vi "Control Type.vi"(11 "Valve in":refnum<class "InterlockControl.lvclass">) -> (2 "Valve Type":string)   [LabVIEW 2020, in "VolatusControl.lvlib" / "InterlockControl.lvclass"]
uses:
  InterlockControl.lvclass
  InterlockControl.lvclass/InterlockControl.ctl
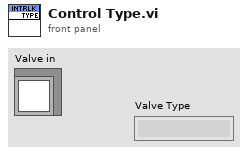
[diagram p1: front panel]
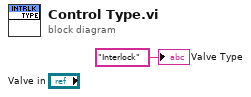
[diagram p0: block diagram]
diagram:
  "Valve Type" <- "Interlock" ("Valve Type")
